vi "Last shot web method.vi"() -> (3 "Shot number":string="Last shot text\ngoes here")   [LabVIEW 2012]
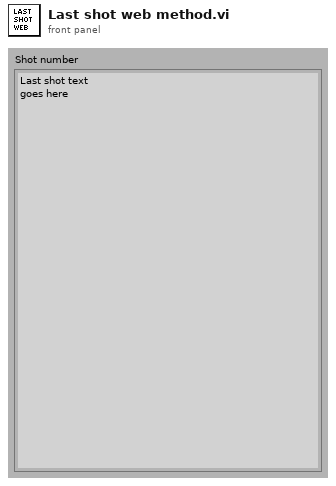
[diagram p1: front panel]
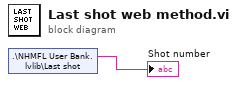
[diagram p0: block diagram]
diagram:
  n1 = shared-variable ".\\NHMFL User Bank.lvlib\\Last shot"() -> (→"Shot number":string)  [unwired: 1 in, 1 out]
